vi "M_ClmnListBox_ItemNames_GET_Test.vi"(7 "Label":string, 8 "error in":errorcluster, 11 "VI Server.RefsCluster":T2) -> (0 "error out":errorcluster, 3 "VI Server.RefsCluster.DUP":T2)   [LabVIEW 2020]
uses:
  VI Server_TypeDefs/VI Server_RefsCluster.ctl
  <vilib>/Utility/miscctls.llb/LVRowAndColumnTypeDef.ctl
panel:
  out "Cell.String":string
  in  "Selected Cell":T1
  in  "Stop Button":bool
  in  "Multicolumn Listbox":i32[](listbox)
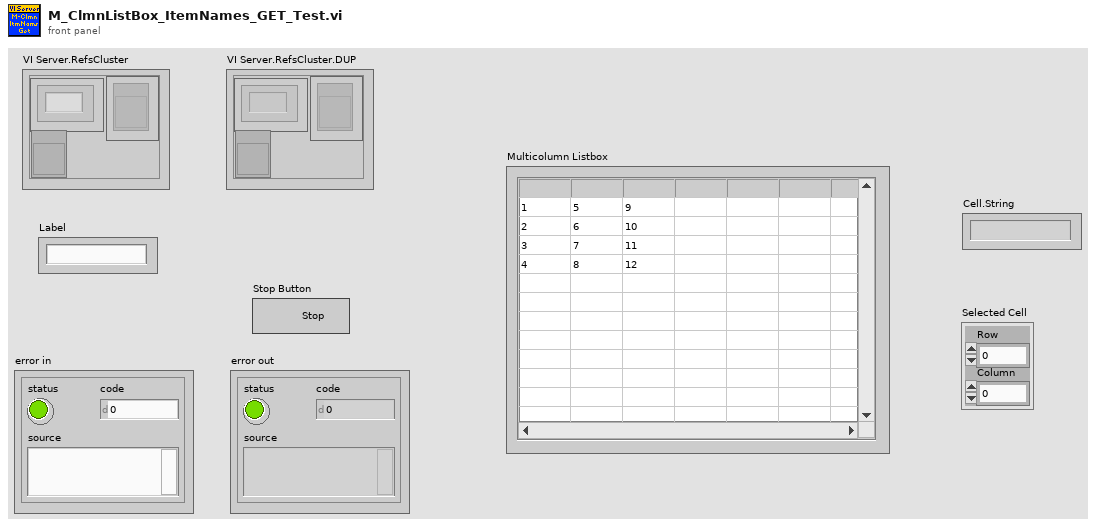
[diagram p1: front panel]
types:
  T1 = typedef "LVRowAndColumnTypeDef.ctl" = cluster{"Row":i32, "Column":i32}
  T2 = typedef "VI Server_RefsCluster.ctl" = cluster{"Labels":string[], "Refs":refnum<vi>[], "VI Ref":refnum<vi>}
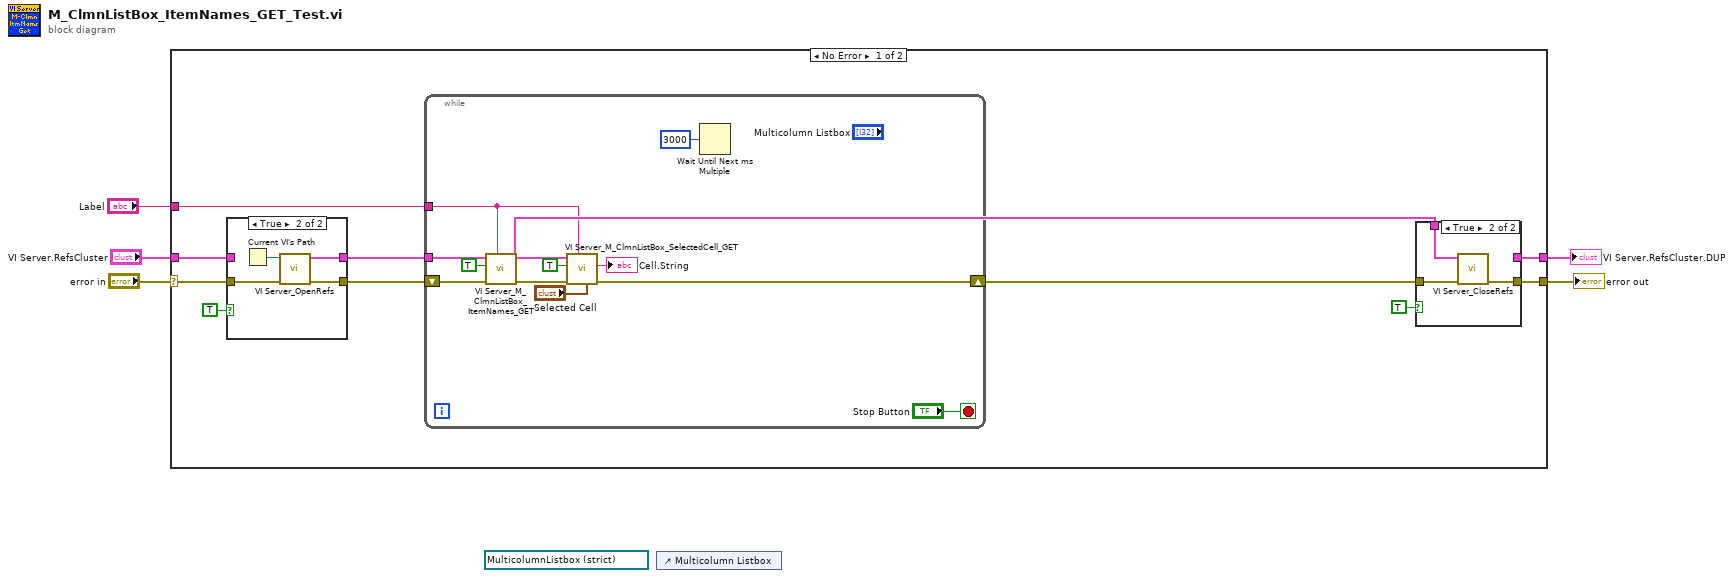
[diagram p0: block diagram]
diagram:
  (unwired) refnum<vi> refnum ("Multicolumn Listbox")
  n1 = case shown="No Error" "error in" {
    selector: "error in" -> [w15 w40]
    tunnel: [w12 w40] -> w4
    tunnel: "VI Server.RefsCluster" -> [w13 w39]
    tunnel: [w10 w39] -> w2
    tunnel: "Label" -> [w6 _]
    frame No Error {
      n2 = case shown="True" TRUE {
        tunnel: w15 -> [w34 w38]
        tunnel: [w34 w36] -> w9
        tunnel: [w33 w35] -> w7
        tunnel: w13 -> [w33 _]
        frame False {
        }
        frame True {
          n3 = Current VI's Path() -> (path=w37:path)
          n4 = call "VI Server_OpenRefs.vi"("error in"=w38, "VI Path"=w37) -> ("error out"=w36:errorcluster, "VI Server.RefsCluster"=w35:T2)  [unwired: 8 in]
        }
      }
      n5 = while {
        tunnel: w7 -> [w26]
        tunnel: w6 -> [w19]
        shift-right: [w21] -> w8
        shift-left: w9 -> [w27]
        stop <- "Stop Button" stop-if-true
        n6 = call "VI Server_M_ClmnListBox_ItemNames_GET.vi"("Label"=w19, "error in"=w27, "SingleInstance"=TRUE, "VI Server.RefsCluster"=w26) -> ("error out"=w22:errorcluster, "VI Server.RefsCluster.DUP"=w20:T2)  [unwired: 1 in, 5 out]
        n7 = call "VI Server_M_ClmnListBox_SelectedCell_GET.vi"("Selected Cell"="Selected Cell", "Label"=w19, "error in"=w22, "SingleInstance"=TRUE, "VI Server.RefsCluster"=w20) -> ("error out"=w21:errorcluster, "Cell.String"=→"Cell.String":string)  [unwired: 3 in, 2 out]
        n8 = Wait Until Next ms Multiple(millisecond multiple=u32 3000) -> ()  [unwired: 1 out]
      }
      n9 = case shown="True" TRUE {
        tunnel: w8 -> [w29 w32]
        tunnel: [w29 w31] -> w12
        tunnel: w7 -> [w28 w30]
        tunnel: [w28 _] -> w10
        frame False {
        }
        frame True {
          n10 = call "VI Server_CloseRefs.vi"("error in"=w32, "VI Server.RefsCluster"=w30) -> ("error out"=w31:errorcluster)  [unwired: 9 in]
        }
      }
    }
    frame Error {
    }
  }
  "VI Server.RefsCluster.DUP" <- w2
  "error out" <- w4
  n11 = control-ref of="Multicolumn Listbox"() -> ()  [unwired: 1 out]
